vi "PublishMqtt.vi"() -> ()   [LabVIEW 2022 SP3]
panel:
  in  "Python path":path
  out "String 5":string
  in  "Subscribe":string
  out "String 2":string
  in  "Numeric 3":dbl
  in  "Numeric 2":dbl
  in  "Numeric":dbl
  in  "publish":string
  in  "module path":path
  in  "Python version":string
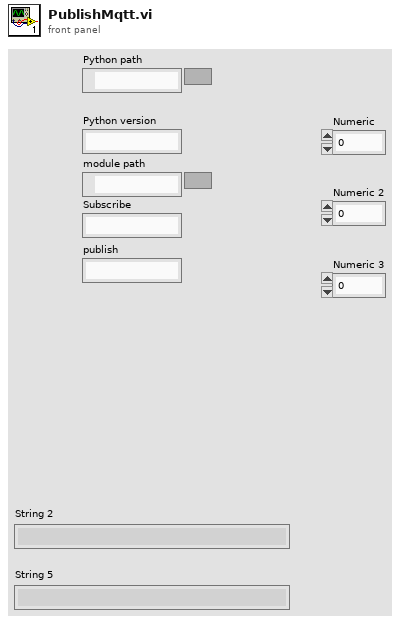
[diagram p1: front panel]
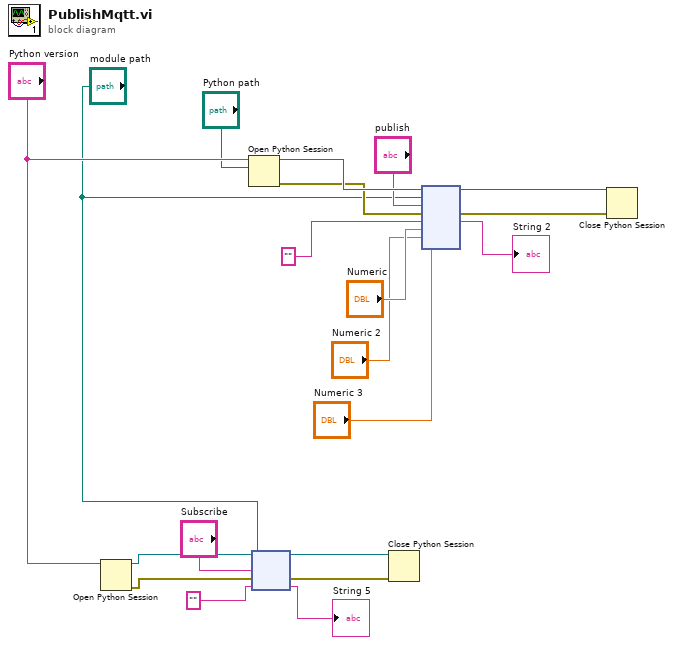
[diagram p0: block diagram]
diagram:
  n1 = Open Python Session(python version="Python version") -> (session out=w11:refnum<k35>, error out=w9:errorcluster)  [unwired: 2 in]
  n2 = Open Python Session(python version="Python version", python path="Python path") -> (session out=w20:refnum<k35>, error out=w14:errorcluster)  [unwired: 1 in]
  n3 = node(w11, "module path", "Subscribe", w9, "") -> (w8:refnum<k35>, w7:errorcluster, →"String 5":string)  [unwired: 2 out]
  n4 = Close Python Session(session in=w8, error in=w7) -> ()  [unwired: 1 out]
  n5 = node(w20, "module path", "publish", w14, "", "Numeric", "Numeric 2", "Numeric 3") -> (w19:refnum<k35>, w13:errorcluster, →"String 2":string)  [unwired: 3 in, 2 out]
  n6 = Close Python Session(session in=w19, error in=w13) -> ()  [unwired: 1 out]
